vi "Pockels Cal-Synthesize initial message.vi"() -> (3 "Message":string)   [LabVIEW 2013]
uses:
  Globals/gl_Calibration globals.vi
  Global Variables/gl_UI Ctrl Refs.vi
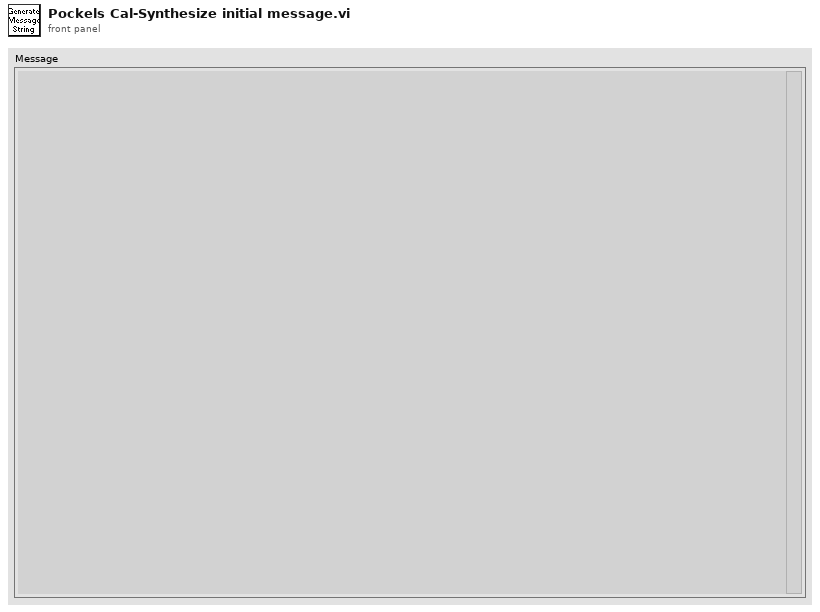
[diagram p1: front panel]
types:
  T1 = typedef "UI ctrl refs cluster.ctl" = cluster{"Top level VI path":path, "Top level VI ref":refnum<vi>, "User menu ref":refnum<k9>, "Sub Panel control":refnum<vi>, "Imaging Param Tab":refnum<vi>, "Occurrence-Start drivers":refnum<k4>, "Occurrence-Speed logging initialised":refnum<k4>, "Occurrence-XYZ stage initialised":refnum<k4>, "Exit button":refnum<vi>, "Status ind":refnum<vi>, "Return to Origin":refnum<vi>, "Speed Logging":refnum<vi>, "Time Lapse":refnum<vi>, "Live Imaging":refnum<vi>, "AOL Z Stack":refnum<vi>, "Motor Z Stack":refnum<vi>, "Funct Acq button":refnum<vi>, "Hard Shutter":refnum<vi>, "Virtual Shutter":refnum<vi>, "Laser Power":refnum<vi>, "AOL Mode":refnum<vi>, "Frame Size":refnum<vi>, "Field of View":refnum<vi>, "Dwell Time":refnum<vi>, "Zoom":refnum<vi>, "AOL Z":refnum<vi>, "Objective":refnum<vi>, "Axis":refnum<vi>, "Paths & Names":refnum<vi>, "Experiment folder path (ind.)":refnum<vi>, "Last State (Ind.)":refnum<vi>, "Laser wavelength ind (nm)":refnum<vi>, "Averages":refnum<vi>, "Angle (degrees)":refnum<vi>, "X centre":refnum<vi>, "Y centre":refnum<vi>, "Plane Mode":refnum<vi>, "# Planes":refnum<vi>, "Z Start":refnum<vi>, "Z Stop":refnum<vi>, "Z Step":refnum<vi>, "PMT 1":refnum<vi>, "PMT 2":refnum<vi>, "Stage XYZ Position":refnum<vi>, "Pockels@Z Start":refnum<vi>, "Pockels@Z Stop":refnum<vi>, "Obtain Z Start":refnum<vi>, "Obtain Z Stop":refnum<vi>, "Live stim.trig.period":refnum<vi>, "Live stim.trig.enable":refnum<vi>, "Funct. Acq. Pockels Modulation":refnum<vi>, "Enable Video Recording":refnum<vi>, "Video Record-Live Imaging":refnum<vi>, "Video Record-Funct acq":refnum<vi>, "AOL Z-stack Chirps Ready (ind)":refnum<vi>, "Center freq ind (nm)":refnum<vi>, "Logging queue (ind)":refnum<vi>, "Back aperture power (ind.)":refnum<vi>, "Power after objective (ind.)":refnum<vi>, "Switch user":refnum<vi>}
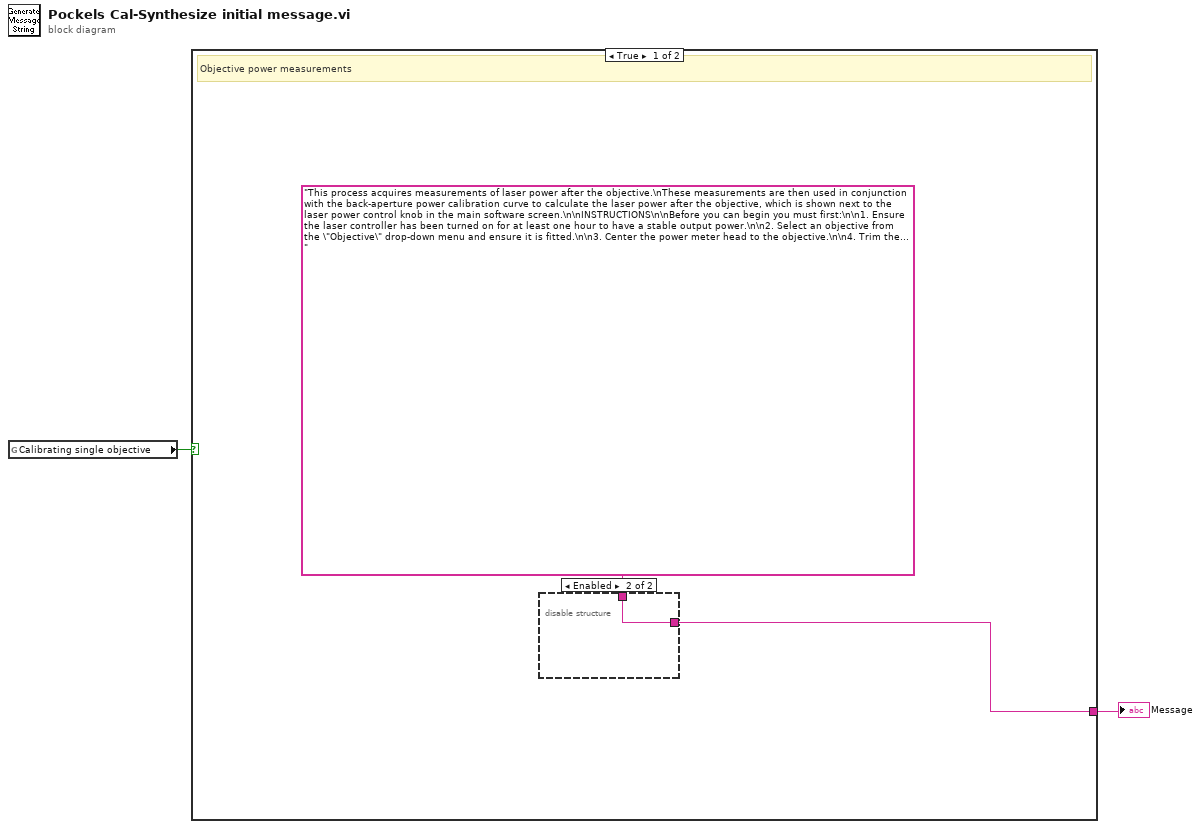
[diagram p0: block diagram]
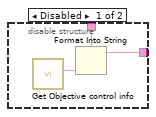
[diagram p2: hidden frame]
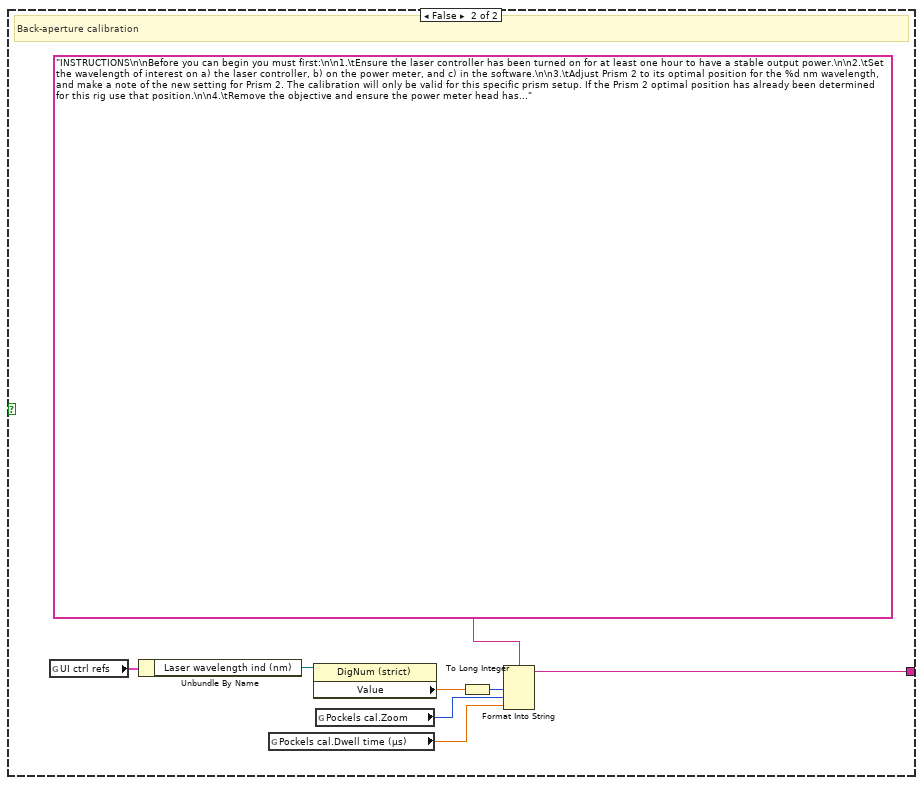
[diagram p3: hidden frame]
diagram:
  n1 = global read "gl_Calibration globals.vi" "Calibrating single objective"() -> (w2:bool)
  n2 = case shown="True" w2 {
    tunnel: [w3 w9] -> w1
    frame True {
      # "Objective power measurements"
      n3 = disable-structure shown="Enabled" {
        disable-tunnel: "This process acquires measurements of laser power after the objective.\nThese measurements are then used in conjunction with the back-aperture power calibration curve to calculate the laser power after the objective, which is shown next to the laser power control knob in the main software screen.\n\nINSTRUCTIONS\n\nBefore you can begin you must first:\n\n1. Ensure the laser controller has been turned on for at least one hour to have a stable output power.\n\n2. Select an objective from the \"Objective\" drop-down menu and ensure it is fitted.\n\n3. Center the power meter head to the objective.\n\n4. Trim the power meter to zero without laser (i.e. no imaging running).\n\t\n5. DO NOT touch the power meter head (it is pyro-electric).\n" ("Message string") -> [w7 w8]
        disable-tunnel: [w5 w8] -> w3
        frame Disabled {
          n4 = call "Get Objective control info.vi"() -> ("Value"=w6:string)  [unwired: 7 in, 4 out]
          n5 = Format Into String(format string=w7, w6) -> (resulting string=w5:string)  [unwired: 2 in, 1 out]
        }
        frame Enabled {
        }
      }
    }
    frame False {
      # "Back-aperture calibration"
      n6 = global read "gl_UI Ctrl Refs.vi" "UI ctrl refs"() -> (w15:T1)
      n7 = Unbundle By Name(w15) -> ("Laser wavelength ind (nm)"=w13:refnum<vi>)
      n8 = global read "gl_Calibration globals.vi" "Pockels cal.Dwell time (µs)"() -> (w11:dbl)
      n9 = property class="DigNum (strict)"(reference=w13) -> ("Value"=w12:dbl)  [unwired: 1 in, 2 out]
      n10 = global read "gl_Calibration globals.vi" "Pockels cal.Zoom"() -> (w16:u8)
      n11 = To Long Integer(number=w12) -> (32bit integer=w14:i32)
      n12 = Format Into String(format string="INSTRUCTIONS\n\nBefore you can begin you must first:\n\n1.\tEnsure the laser controller has been turned on for at least one hour to have a stable output power.\n\n2.\tSet the wavelength of interest on a) the laser controller, b) on the power meter, and c) in the software.\n\n3.\tAdjust Prism 2 to its optimal position for the %d nm wavelength, and make a note of the new setting for Prism 2. The calibration will only be valid for this specific prism setup. If the Prism 2 optimal position has already been determined for this rig use that position.\n\n4.\tRemove the objective and ensure the power meter head has been centred.\n\n5.\tTrim the power meter to zero without laser (i.e. no imaging running).\n\t\n6.\tDO NOT touch the power meter head (it is pyro-electric).\n\nAre you ready to start the Pockels calibration wizard?\n(see notes below)\n\n\n\nNOTES:\n\na) The calibration curve generated at the end of this process will be specific to the \"Laser wavelength\" currently selected. Run the calibration wizard again for each wavelength of interest. Each new calibration curve is added to the same calibration file by default.\n\nb) The zoom and dwell time will be automatically set to %dx and %.1fµs respectively. \nThese values can be changed through the System Configuration window but you must use the same values across all calibration curves (i.e. one curve per laser wavelength of interest) you add within a single pockels calibration file.\n\nc) During normal operation the software automatically loads the correct calibration for the specified wavelength if one exists. Otherwise it will generate a warning message and it will use a default calibration just to allow the rig to run.\n\nd) During the calibration process keep in mind that it is normal for the measured power to saturate and even reduce a little after around 1.5V.\n\ne) At the end of the calibration process you can chose to save the calibration curve to a new file.\n\n\nAre you ready to start the Pockels calibration wizard?\n" ("Message string"), w14, w16, w11) -> (resulting string=w9:string)  [unwired: 2 in, 1 out]
    }
  }
  "Message" <- w1
